vi "Transducer Calibration.vi"() -> ()   [LabVIEW 2016]
panel:
  in  "Comment":string
  in  "Filename":path=path "test.tdms"
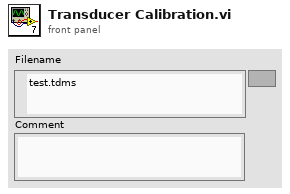
[diagram p1: front panel]
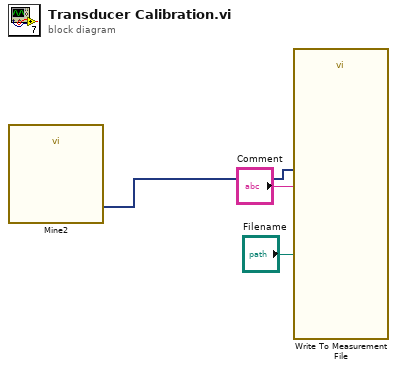
[diagram p0: block diagram]
diagram:
  n1 = call "Mine2"() -> ("data"=w1:dynamicdata)  [unwired: 17 in, 2 out]
  n2 = call "Write To Measurement File"("Signals"=w1, "Filename"="Filename", "Comment"="Comment") -> ()  [unwired: 14 in, 3 out]
